vi "Get BuildSpec Names.vi"(11 "LabVIEW Build Script in":refnum<class "LabVIEW Build Script.lvclass">) -> (3 "BuildSpecs":string[](array[string]))   [LabVIEW 2021, in "LabVIEW Build Script.lvclass"]
uses:
  LabVIEW Build Script.lvclass
  LabVIEW Build Script.lvclass/LabVIEW Build Script.ctl
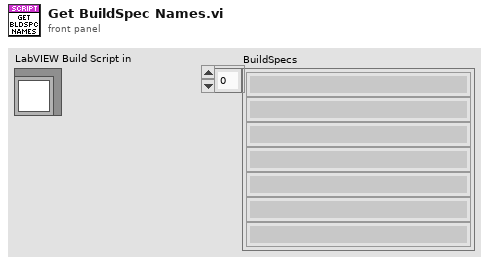
[diagram p1: front panel]
types:
  T1 = typedef "LV Scripting Utilities.lvlib/BuildSpec Map.ctl" = map{string, refnum<vi>}
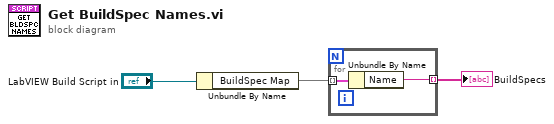
[diagram p0: block diagram]
diagram:
  n1 = Unbundle By Name("LabVIEW Build Script in") -> ("BuildSpec Map"=w2:T1)
  n2 = for {
    tunnel: w2 -> [w5] mode=indexing
    tunnel: [w4] -> w1 mode=indexing
    n3 = Unbundle By Name(w5) -> ("Name"=w4:string)
  }
  "BuildSpecs" <- w1
